vi "holdGalvos.vi"() -> ()   [LabVIEW 2017]
doc: "This example demonstrates how to generate a user-defined voltage using the analog output of a DAQ device."
uses:
  <vilib>/Utility/error.llb/DialogType.ctl
  <vilib>/DAQmx/write.llb/DAQmx Write (Analog 1D DBL NChan 1Samp).vi
  <vilib>/DAQmx/create/channels.llb/DAQmx Create Channel (AO-Voltage-Basic).vi
  <vilib>/DAQmx/miscellaneous.llb/DAQmx Fill In Error Info.vi
panel:
  out "Y (deg)":dbl
  out "X (deg)":dbl
  in  "Y (V)":dbl min=-5.0 max=5.0
  in  "X (V)":dbl min=-5.0 max=5.0
  in  "Stop":bool
  in  "Max Voltage":dbl=5.0
  in  "Min Voltage":dbl=-5.0
  in  "Physical Channel(s)":tag="Dev1/ao0:1"
  # "Channel Settings"
  # "Output"
  # "Run, set X and Y to 0V during sample arm alignment."
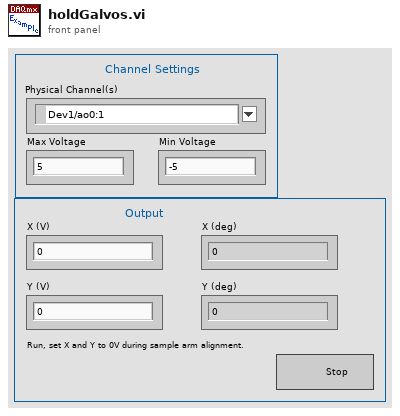
[diagram p1: front panel]
types:
  T1 = typedef "DialogType.ctl" = u16
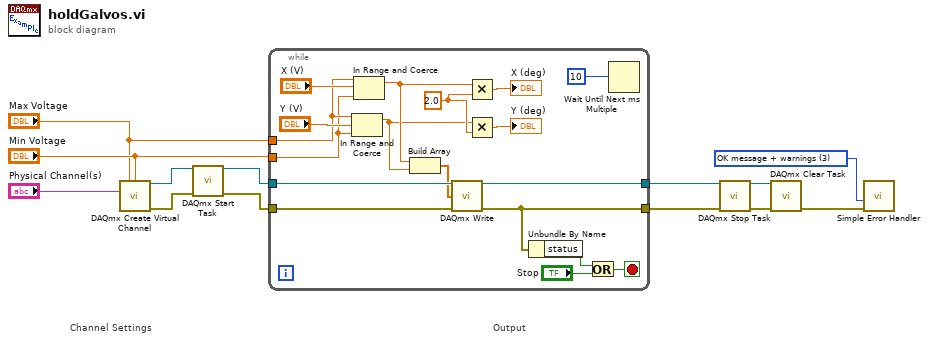
[diagram p0: block diagram]
diagram:
  w3 = T1 3 items=["no dialog", "OK message", "continue or stop message", "OK message + warnings", "continue/stop + warnings"] ("type of dialog (OK msg:1)")
  # "Output"
  # "Channel Settings"
  n1 = call-poly <vilib>:"DAQmx Create Virtual Channel.vi"("maximum value"="Max Voltage", "minimum value"="Min Voltage", "physical channels"="Physical Channel(s)") -> ("task out"=w11:refnum<k21>, "error out"=w10:errorcluster)  [unwired: 11 in]
  n2 = call <vilib>:"DAQmx Start Task.vi"("task/channels in"=w11, "error in"=w10) -> ("task out"=w9:refnum<k21>, "error out"=w8:errorcluster)  [unwired: 12 in]
  n3 = while {
    tunnel: w9 -> [w31]
    tunnel: w8 -> [w30]
    tunnel: [w25] -> w6
    tunnel: [w29] -> w7
    tunnel: "Min Voltage" -> [w14]
    tunnel: "Max Voltage" -> [w15]
    stop <- w24 stop-if-true
    w20 = 2.0 ("y")
    n4 = In Range and Coerce(upper limit=w15, x="Y (V)", lower limit=w14) -> (coerced(x)=w16:dbl)  [unwired: 1 out]
    n5 = In Range and Coerce(upper limit=w15, x="X (V)", lower limit=w14) -> (coerced(x)=w19:dbl)  [unwired: 1 out]
    n6 = Build Array(w19, w16) -> (w23:dbl[])
    n7 = call-poly <vilib>:"DAQmx Write.vi"("task/channels in"=w31, "data"=w23, "error in"=w30) -> ("task out"=w29:refnum<k21>, "error out"=w25:errorcluster)  [unwired: 10 in, 1 out]
    n8 = Multiply(x=w19, y=w20) -> (x*y=→"X (deg)":dbl)
    n9 = Multiply(x=w16, y=w20) -> (x*y=→"Y (deg)":dbl)
    n10 = Unbundle By Name(w25) -> ("status"=w27:bool)
    n11 = Or(x=w27, y="Stop") -> (x .or. y?=w24:bool)
    n12 = Wait Until Next ms Multiple(millisecond multiple=u32 10) -> ()  [unwired: 1 out]
  }
  n13 = call <vilib>:"DAQmx Stop Task.vi"("task/channels in"=w7, "error in"=w6) -> ("task out"=w5:refnum<k21>, "error out"=w4:errorcluster)  [unwired: 12 in]
  n14 = call <vilib>:"DAQmx Clear Task.vi"("task in"=w5, "error in"=w4) -> ("error out"=w13:errorcluster)  [unwired: 13 in]
  n15 = call <vilib>:"Simple Error Handler.vi"("type of dialog (OK msg:1)"=w3, "error in (no error)"=w13) -> ()  [unwired: 3 in, 5 out]
